vi "Obtain Request Events.vi"(8 "error in":errorcluster, 10 "Create New? (F)":bool) -> (0 "error out":errorcluster, 2 "MainPanel Request Events":T1)   [LabVIEW 2022 SP3, in "MainPanel.lvlib"]
doc: "This VI Obtains/Creates the Requests events that will be used for other modules to communicate with the module that owns this VI. These Requests events will be accessed only via Public API methods for this module.\n\n<b>NOTE</b>: The contents of this VI are automatically generated and modified by the <b>Tools > DQMH Consortium > DQMH</b> utilities. Consider using those utilities instead of making your own modifications to this VI.\n_____\nBased on DQMH Project Template 7.0.1.1316."
uses:
  MainPanel.lvlib
  Request Events--cluster.ctl
  Stop Argument--cluster.ctl
  Do Something Argument--cluster.ctl
  Do Something Else Argument--cluster.ctl
  Do Something Else and Wait for Reply Argument--cluster.ctl
  Do Something Else and Wait (Reply Payload)--cluster.ctl
  Show Panel Argument--cluster.ctl
  Hide Panel Argument--cluster.ctl
  Get Module Execution Status Argument--cluster.ctl
  Show Diagram Argument--cluster.ctl
  Prepare Argument--cluster.ctl
  Configure Argument--cluster.ctl
  Request UI Display Argument--cluster.ctl
  Framework/UI Manager/Module Display Scenarios.ctl
  Request UI Display (Reply Payload)--cluster.ctl
  Framework/UI Manager/UI Manager.lvlib
  Update UI Argument--cluster.ctl
panel:
  # "NOTE: The contents of this VI are automatically generated and modified by the Tools > DQMH Consortium > DQMH utilities. Consider using those utilities instead of making your own modifications to this VI."
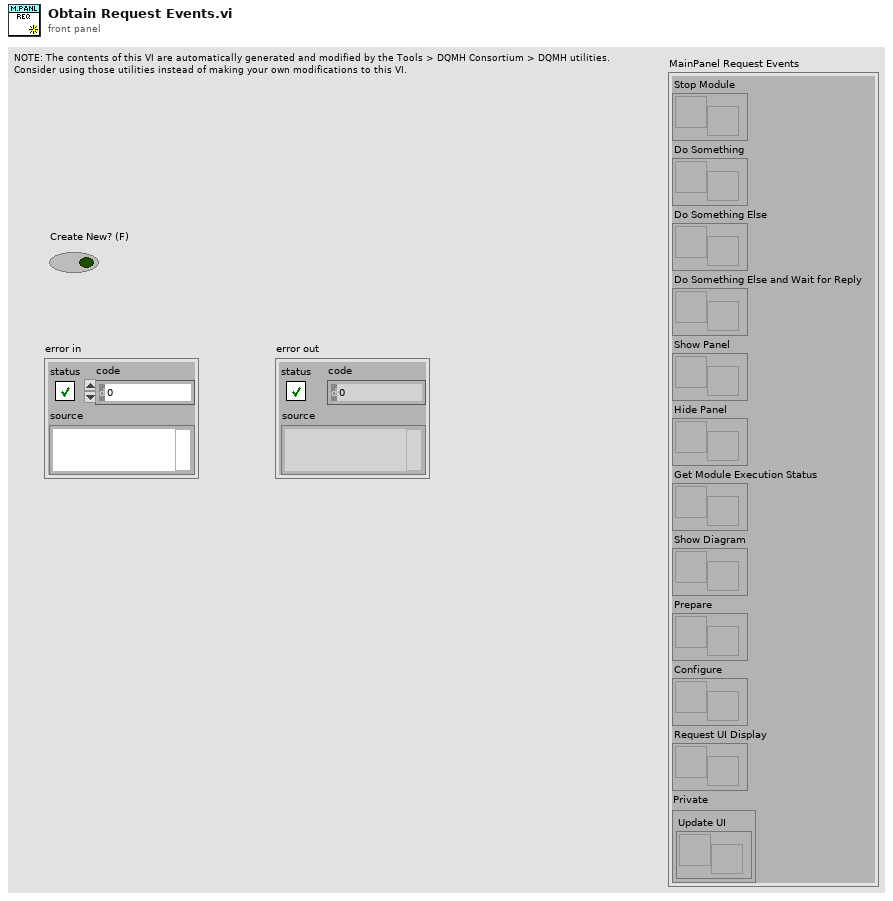
[diagram p1: front panel]
types:
  T1 = typedef "MainPanel.lvlib/Request Events--cluster.ctl" = cluster{"Stop Module":refnum<user-event>, "Do Something":refnum<user-event>, "Do Something Else":refnum<user-event>, "Do Something Else and Wait for Reply":refnum<user-event>, "Show Panel":refnum<user-event>, "Hide Panel":refnum<user-event>, "Get Module Execution Status":refnum<user-event>, "Show Diagram":refnum<user-event>, "Prepare":refnum<user-event>, "Configure":refnum<user-event>, "Request UI Display":refnum<user-event>, "Private":cluster{"Update UI":refnum<user-event>}}
  T2 = typedef "MainPanel.lvlib/Update UI Argument--cluster.ctl" = cluster{"Update":bool}
  T3 = typedef "MainPanel.lvlib/Request UI Display Argument--cluster.ctl" = cluster{"Scenario":T4, "Wait Notifier":refnum<notifier>, "wait for reply":bool}
  T4 = typedef "UI Manager.lvlib/Module Display Scenarios.ctl" = enum16{"Stand-Alone", "Managed"}
  T5 = typedef "MainPanel.lvlib/Configure Argument--cluster.ctl" = cluster{"Boolean":bool}
  T6 = typedef "MainPanel.lvlib/Prepare Argument--cluster.ctl" = cluster{"Boolean":bool}
  T7 = typedef "MainPanel.lvlib/Hide Panel Argument--cluster.ctl" = cluster{"Hide Panel?":bool}
  T8 = typedef "MainPanel.lvlib/Show Panel Argument--cluster.ctl" = cluster{"Show Panel?":bool}
  T9 = typedef "MainPanel.lvlib/Show Diagram Argument--cluster.ctl" = cluster{"Debug?":bool}
  T10 = typedef "MainPanel.lvlib/Get Module Execution Status Argument--cluster.ctl" = cluster{"Running?":bool}
  T11 = typedef "MainPanel.lvlib/Do Something Else and Wait for Reply Argument--cluster.ctl" = cluster{"Do Something Else Msg":string, "X":dbl, "Wait Notifier":refnum<notifier>, "wait for reply":bool}
  T12 = typedef "MainPanel.lvlib/Do Something Else Argument--cluster.ctl" = cluster{"Do Something Else Msg":string, "X":dbl}
  T13 = typedef "MainPanel.lvlib/Do Something Argument--cluster.ctl" = cluster{"Do Something Msg":string}
  T14 = typedef "MainPanel.lvlib/Stop Argument--cluster.ctl" = cluster{"Origin":string, "Exit via Stop Module Req?":bool, "Wait for Module to stop?":bool}
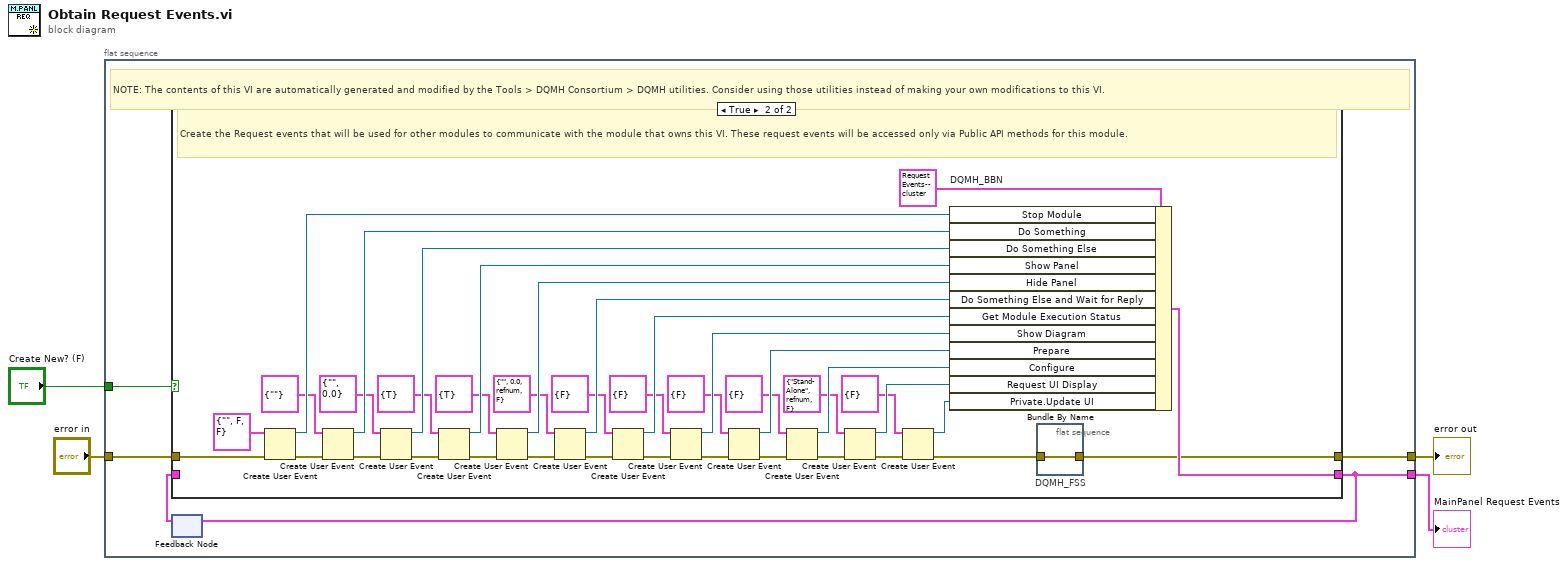
[diagram p0: block diagram]
diagram:
  n1 = flat-sequence {
    tunnel: [w9] -> w4
    tunnel: "error in" -> [w8]
    tunnel: [w6] -> w2
    tunnel: "Create New? (F)" -> [w5]
    frame #0 {
      # "NOTE: The contents of this VI are automatically generated and modified by the Tools > DQMH Consortium > DQMH utilities. Consider using those utilities instead of making your own modifications to this VI."
      n2 = feedback #1() -> (w7:T1)  [unwired: 1 in]
      n3 = case shown="True" w5 {
        tunnel: [w10 w32] -> w9
        tunnel: w8 -> [w10 w51]
        tunnel: [w11 w48] -> w6
        tunnel: w7 -> [w11 _]
        frame False {
          # "Obtain the Request events that were created in a previous call to this VI."
        }
        frame True {
          # "Create the Request events that will be used for other modules to communicate with the module that owns this VI. These request events will be accessed only via Public API methods for this module."
          n4 = Create User Event(user event datatype=T14 {"Origin"="", "Exit via Stop Module Req?"=FALSE, "Wait for Module to stop?"=FALSE} ("Stop Argument"), error in=w51) -> (user event=w49:refnum<user-event>, error out=w45:errorcluster)
          n5 = Create User Event(user event datatype=T13 {"Do Something Msg"=""} ("Do Something Argument"), error in=w45) -> (user event=w44:refnum<user-event>, error out=w43:errorcluster)
          n6 = Create User Event(user event datatype=T12 {"Do Something Else Msg"="", "X"=0.0} ("Do Something Else Argument"), error in=w43) -> (user event=w41:refnum<user-event>, error out=w40:errorcluster)
          n7 = Create User Event(user event datatype=T8 {"Show Panel?"=TRUE} ("Show Panel Argument"), error in=w40) -> (user event=w39:refnum<user-event>, error out=w38:errorcluster)
          n8 = Create User Event(user event datatype=T7 {"Hide Panel?"=TRUE} ("Hide Panel Argument"), error in=w38) -> (user event=w37:refnum<user-event>, error out=w36:errorcluster)
          n9 = Create User Event(user event datatype=T11 {"Do Something Else Msg"="", "X"=0.0, "Wait Notifier"=refnum, "wait for reply"=FALSE} ("Do Something Else and Wait for Reply Argument"), error in=w36) -> (user event=w35:refnum<user-event>, error out=w33:errorcluster)
          n10 = Create User Event(user event datatype=T10 {"Running?"=FALSE} ("Get Module Execution Status Argument"), error in=w33) -> (user event=w30:refnum<user-event>, error out=w31:errorcluster)
          n11 = Create User Event(user event datatype=T9 {"Debug?"=FALSE} ("Show Diagram Argument"), error in=w31) -> (user event=w27:refnum<user-event>, error out=w28:errorcluster)
          n12 = Create User Event(user event datatype=T6 {"Boolean"=FALSE} ("Prepare Argument"), error in=w28) -> (user event=w22:refnum<user-event>, error out=w23:errorcluster)
          n13 = Create User Event(user event datatype=T5 {"Boolean"=FALSE} ("Configure Argument"), error in=w23) -> (user event=w19:refnum<user-event>, error out=w20:errorcluster)
          n14 = Create User Event(user event datatype=T3 {"Scenario"=enum."Stand-Alone", "Wait Notifier"=refnum, "wait for reply"=FALSE} ("Request UI Display Argument"), error in=w20) -> (user event=w16:refnum<user-event>, error out=w17:errorcluster)
          n15 = Create User Event(user event datatype=T2 {"Update"=FALSE} ("Update UI Argument"), error in=w17) -> (user event=w13:refnum<user-event>, error out=w14:errorcluster)
          n16 = Bundle By Name "DQMH_BBN"(cluster=T1 {"Stop Module"=refnum, "Do Something"=refnum, "Do Something Else"=refnum, "Do Something Else and Wait for Reply"=refnum, "Show Panel"=refnum, "Hide Panel"=refnum, "Get Module Execution Status"=refnum, "Show Diagram"=refnum, "Prepare"=refnum, "Configure"=refnum, "Request UI Display"=refnum, "Private"={"Update UI"=refnum}} ("output cluster"), "Stop Module"=w49, "Do Something"=w44, "Do Something Else"=w41, "Show Panel"=w39, "Hide Panel"=w37, "Do Something Else and Wait for Reply"=w35, "Get Module Execution Status"=w30, "Show Diagram"=w27, "Prepare"=w22, "Configure"=w19, "Request UI Display"=w16, "Private.Update UI"=w13) -> (w48:T1)
          n17 = flat-sequence "DQMH_FSS" {
            tunnel: w14 -> [w52]
            tunnel: [w52] -> w32
            frame #0 {
            }
          }
        }
      }
      n18 = feedback-in #1(w6) -> ()
    }
  }
  "MainPanel Request Events" <- w2
  "error out" <- w4
